vi "Actor Core.vi"(8 "error in":errorcluster, 11 "Nested in":refnum<class "Lock-In Remote Actor.lvclass">) -> (0 "error out":errorcluster, 3 "Actor out":refnum<class "Actor.lvclass">)   [LabVIEW 2023, in "Lock-In Remote Actor.lvlib" / "Lock-In Remote Actor.lvclass"]
doc: "(<B>Filename</B>: Actor Framework.lvlib:Actor.lvclass:Actor Core.vi)\n\nReceives messages to the actor, reacts to them, and initiates any error handling that may shut the actor down.\n\nDescendant classes may override this VI to append parallel tasks for the actor to complete while it handles messages. Overrides use the Call Parent Method node."
uses:
  Lock-In Remote Actor.lvclass
  C:/Program Files/National Instruments/LabVIEW 2023/vi.lib/ActorFramework/Actor/Actor.lvclass
  <vilib>/ActorFramework/Actor/Actor.lvclass
  <vilib>/ni/Actors/Network Endpoint Actors/Notifying Nested Endpoint/Notifying Nested Endpoint.lvclass
  C:/Program Files/National Instruments/LabVIEW 2023/vi.lib/ni/Actors/Network Endpoint Actors/Network Endpoint/Network Endpoint/Network Endpoint.lvclass
  MSS Remote Actor/MSS Remote Actor.lvclass
  <vilib>/ActorFramework/Actor/Actor.lvclass/Actor.ctl
  <vilib>/ActorFramework/Message Enqueuer/Message Enqueuer.lvclass/Message Enqueuer.ctl
  Lock-In Remote Actor.lvclass/Lock-In Remote Actor.ctl
  <vilib>/ni/Actors/Network Endpoint Actors/Network Endpoint/Network Endpoint/Network Endpoint.lvclass/Network Endpoint.ctl
  <vilib>/ActorFramework/Message Enqueuer/Init from Existing Queue.vi
  <vilib>/ActorFramework/Message Enqueuer/Enqueue.vi
  <vilib>/ActorFramework/Stop Msg/Stop Msg.lvclass
  C:/Program Files/National Instruments/LabVIEW 2023/vi.lib/ActorFramework/Message/Message.lvclass
  <vilib>/ActorFramework/Message Priority Queue/Priority Enqueue.vi
  <vilib>/Utility/error.llb/Error Cluster From Error Code.vi
  <vilib>/ActorFramework/Message Enqueuer/Message Enqueuer.lvclass
  <vilib>/ni/Actors/Network Endpoint Actors/Network Endpoint/Network Endpoint/Network Endpoint.lvclass
panel:
  out "Excitation":T1
  out "Connected":bool
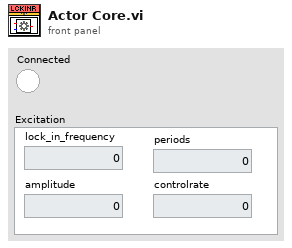
[diagram p1: front panel]
types:
  T1 = cluster{"lock_in_frequency":dbl, "amplitude":dbl, "periods":dbl, "controlrate":dbl}
  T2 = cluster{"Stop":refnum<user-event>, "Connected":refnum<user-event>, "Excitation":refnum<user-event>}
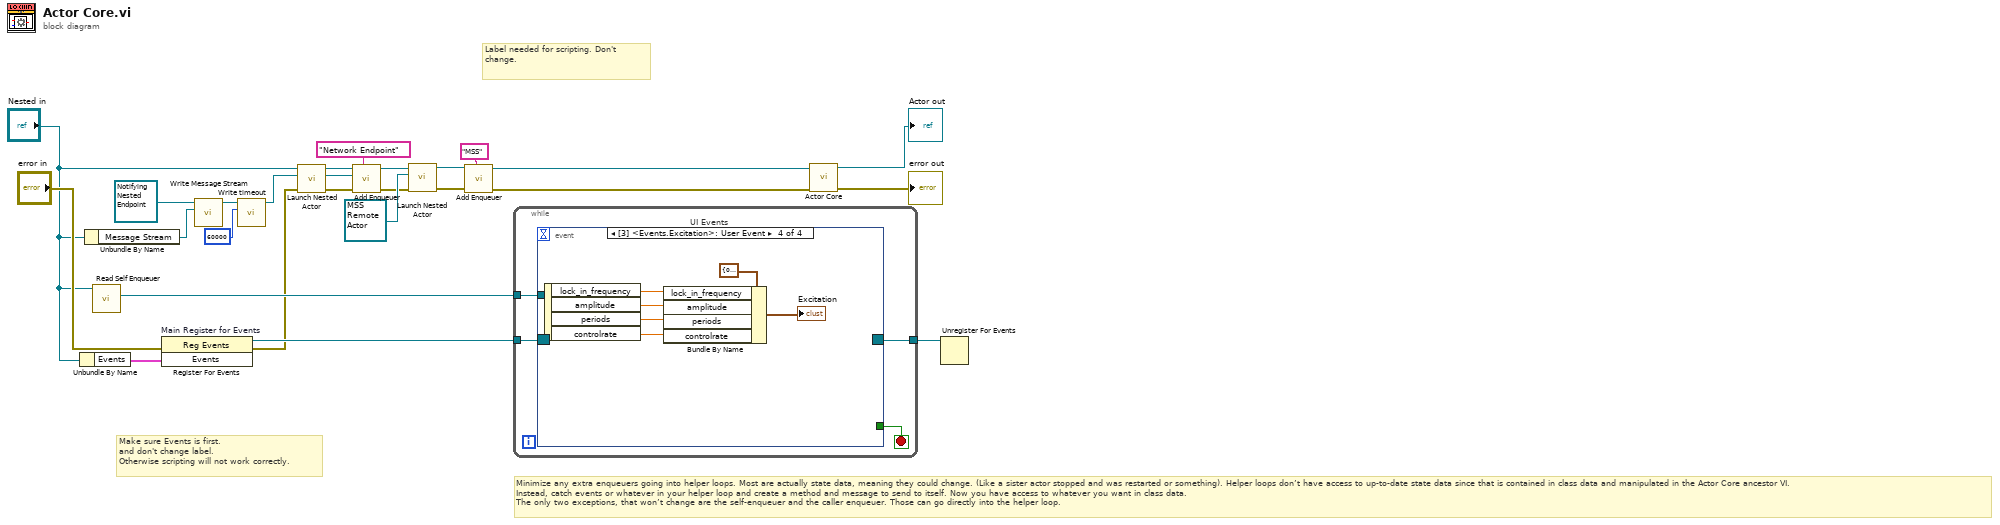
[diagram p0: block diagram]
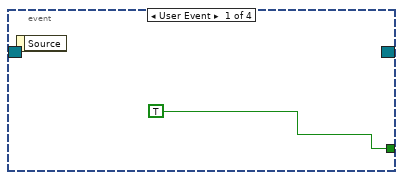
[diagram p2: hidden frame]
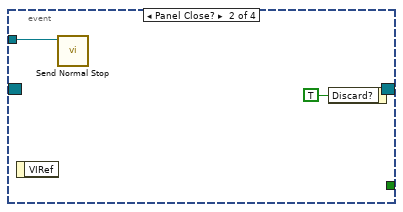
[diagram p3: hidden frame]
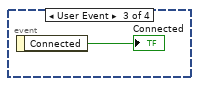
[diagram p4: hidden frame]
diagram:
  # "Minimize any extra enqueuers going into helper loops. Most are actually state data, meaning they could change. (Like a sister actor stopped and was restarted or something). Helper loops don’t have access to up-to-date state data since that is contained in class data and manipulated in the Actor Core ancestor VI.\nInstead, catch events or whatever in your helper loop and create a method and message to send to itself. Now you have access to whatever you want in class data.\nThe only two exceptions, that won’t change are the self-enqueuer and the caller enqueuer. Those can go directly into the helper loop."
  # "Label needed for scripting. Don't change."
  # "Make sure Events is first.\nand don't change label.\nOtherwise scripting will not work correctly."
  n1 = Unbundle By Name("Nested in") -> ("Events"=w23:T2)
  n2 = Unbundle By Name("Nested in") -> ("Message Stream"=w16:refnum<class "Message Stream.lvclass">)
  n3 = call <vilib>:"Read Self Enqueuer.vi"("Actor"="Nested in") -> ("Self Enqueuer"=w21:refnum<class "Message Enqueuer.lvclass">)  [unwired: 10 in]
  n4 = register-events "Main Register for Events"(error in="error in", w23) -> (reference out=w24:refnum<event-registration>, error out=w15:errorcluster)  [unwired: 1 in]
  n5 = call <vilib>:"Write Message Stream.vi"("Message Stream"=w16, "Network Endpoint in"=refnum<class "Notifying Nested Endpoint.lvclass"> refnum ("Notifying Nested Endpoint.lvclass")) -> ("Network Endpoint out"=w18:refnum<class "Notifying Nested Endpoint.lvclass">)  [unwired: 9 in]
  n6 = call <vilib>:"Write timeout.vi"("timeout"=60000, "Network Endpoint in"=w18) -> ("Network Endpoint out"=w13:refnum<class "Notifying Nested Endpoint.lvclass">)  [unwired: 9 in]
  n7 = call <vilib>:"Launch Nested Actor.vi"("error in (no error)"=w15, "Nested Actor"=w13, "Caller Actor in"="Nested in") -> ("error out"=w12:errorcluster, "Nested Actor's Enqueuer"=w7:refnum<class "Message Enqueuer.lvclass">, "Caller Actor out"=w9:refnum<class "Lock-In Remote Actor.lvclass">)  [unwired: 6 in]
  n8 = call "Add Enqueuer.vi"("Enqueuer Ident"="Network Endpoint", "error in (no error)"=w12, "Nested Actor's Enqueuer"=w7, "Lock-In Remote Actor in"=w9) -> ("error out"=w10:errorcluster, "Lock-In Remote Actor out"=w8:refnum<class "Lock-In Remote Actor.lvclass">)  [unwired: 6 in]
  n9 = call <vilib>:"Launch Nested Actor.vi"("error in (no error)"=w10, "Nested Actor"=refnum<class "MSS Remote Actor.lvclass"> refnum ("MSS Remote Actor.lvlib:MSS Remote Actor.lvclass"), "Caller Actor in"=w8) -> ("error out"=w4:errorcluster, "Caller Actor out"=w5:refnum<class "Lock-In Remote Actor.lvclass">)  [unwired: 6 in, 1 out]
  n10 = call "Add Enqueuer.vi"("Enqueuer Ident"="MSS", "error in (no error)"=w4, "Lock-In Remote Actor in"=w5) -> ("error out"=w2:errorcluster, "Lock-In Remote Actor out"=w3:refnum<class "Lock-In Remote Actor.lvclass">)  [unwired: 7 in]
  n11 = while {
    tunnel: w24 -> [w30]
    tunnel: [w28] -> w22
    tunnel: w21 -> [w27]
    stop <- w29 stop-if-true
    n12 = event "UI Events" shown="[3] <Events.Excitation>: User Event" {
      selector: w30 -> [_ _ _ _]
      dyn-events: [_ _ _ _] -> w28
      timeout: _ -> [_ _ _ _]
      tunnel: [TRUE _ _ _] -> w29
      tunnel: w27 -> [_ w32 _ _]
      event User Event {
        n13 = event-data() -> ()  [unwired: 1 in, 1 out]
      }
      event Panel Close? {
        n14 = event-data() -> ()  [unwired: 1 in, 1 out]
        n15 = call <vilib>:"Send Normal Stop.vi"("Message Enqueuer"=w32) -> ()  [unwired: 10 in, 1 out]
        n16 = event-data("Discard?"=TRUE) -> ()  [unwired: 1 in, 1 out]
      }
      event User Event {
        n17 = event-data() -> ("Connected"=→"Connected":bool)  [unwired: 1 in]
      }
      event User Event {
        n18 = event-data() -> ("lock_in_frequency"=w38:dbl, "amplitude"=w37:dbl, "periods"=w36:dbl, "controlrate"=w35:dbl)  [unwired: 1 in]
        n19 = Bundle By Name(cluster=T1 {"lock_in_frequency"=0.0, "amplitude"=0.0, "periods"=0.0, "controlrate"=0.0} ("Excitation"), "lock_in_frequency"=w38, "amplitude"=w37, "periods"=w36, "controlrate"=w35) -> (→"Excitation":T1)
      }
    }
  }
  n20 = call-parent "Actor Core.vi"("error in"=w2, "Actor in"=w3) -> ("error out"=→"error out":errorcluster, "Actor out"=→"Actor out":refnum<class "Actor.lvclass">)  [unwired: 8 in]
  n21 = Unregister For Events(event registration refnum=w22) -> ()  [unwired: 1 in, 1 out]
